vi "get_movie_start_time.vi"(8 "error in (no error)":errorcluster, 11 "ImageCollection.lvclass in":refnum<class "ImageCollection.lvclass">) -> (0 "error out":errorcluster, 2 "movie start":timestamp, 3 "ImageCollection.lvclass out":refnum<class "ImageCollection.lvclass">)   [LabVIEW 2010, in "ImageCollection.lvclass"]
uses:
  ImageCollection.lvclass
  add_mode_enum.ctl
  Image/Image/Image.lvclass
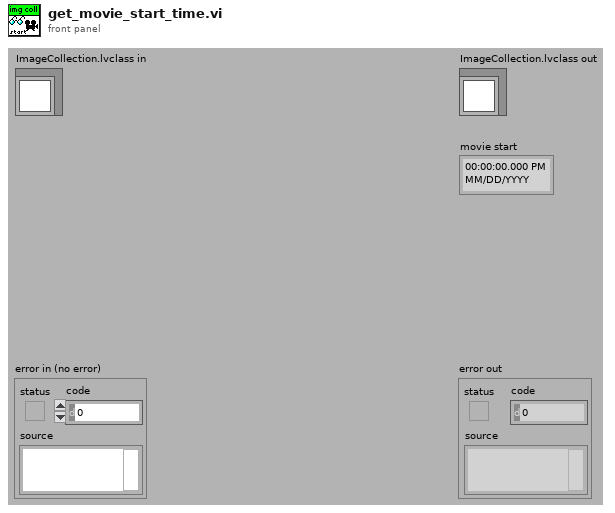
[diagram p1: front panel]
types:
  T1 = typedef "ImageCollection.lvclass/add_mode_enum.ctl" = enum16{"instance", "copy"}
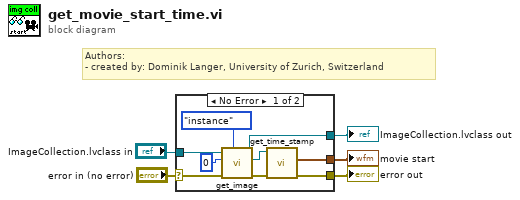
[diagram p0: block diagram]
diagram:
  # "Authors: \n- created by: Dominik Langer, University of Zurich, Switzerland"
  n1 = case shown="No Error" "error in (no error)" {
    selector: "error in (no error)" -> [w7 w15]
    tunnel: [w6 w15] -> w4
    tunnel: [w9 w16] -> w2
    tunnel: "ImageCollection.lvclass in" -> [w10 w16]
    tunnel: [w8 _] -> w1
    frame No Error {
      n2 = call-dynamic "get_image.vi"("get image as..."=add_mode_enum."instance", "error in (no error)"=w7, "index"=0, "ImageCollection in"=w10) -> ("error out"=w12:errorcluster, "Image.lvclass"=w11:refnum<class "Image.lvclass">, "ImageCollection out"=w9:refnum<class "ImageCollection.lvclass">)  [unwired: 5 in]
      n3 = call-dynamic "get_time_stamp.vi"("error in (no error)"=w12, "Image.lvclass in"=w11) -> ("error out"=w6:errorcluster, "timestamp"=w8:timestamp)  [unwired: 7 in, 1 out]
    }
    frame Error {
    }
  }
  "error out" <- w4
  "ImageCollection.lvclass out" <- w2
  "movie start" <- w1
